vi "ClearWarning.vi"(9 "Error in":errorcluster) -> (1 "Error out":errorcluster)   [LabVIEW 2017, in "GPError.lvlib"]
doc: "Clears any warning on <B>Error in</B> but leaves any error.\n\nThis VI supports appended errors, clearing all warnings while leaving any errors.\n\nThis VI is inlined.\n\nSteen Schmidt\nGPower\n18/7 2013"
uses:
  GPError.lvlib
  Append/AppendMulti.vi
panel:
  # "Copyright © 2013\nSteen Schmidt, GPower\nSee enclosed license file for terms and conditions"
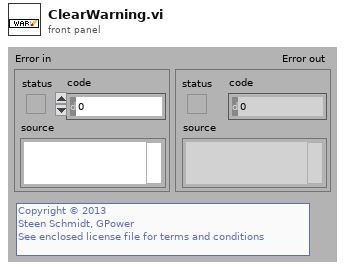
[diagram p1: front panel]
types:
  T1 = typedef "GPError.lvlib/ErrorType.ctl" = enum16{"No Error", "Error", "Warning", "Appended errors", "Appended warnings", "Appended mixed"}
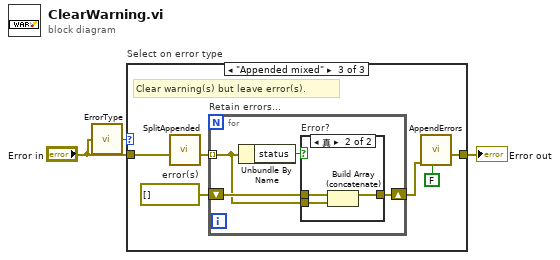
[diagram p0: block diagram]
diagram:
  n1 = call "ErrorType.vi"("Error in"="Error in") -> ("Error type"=w1:T1)  [unwired: 4 in]
  n2 = case "Select on error type" shown="\"Appended mixed\"" w1 {
    tunnel: "Error in" -> [w4 _ w10]
    tunnel: [w4 _ w6] -> w3
    frame "No Error", "Error", "Appended errors" {
      # "Leave 'No error' or error(s)."
    }
    frame "Warning", "Appended warnings" {
      # "Clear warning(s)."
    }
    frame "Appended mixed" {
      w8 = errorcluster[] []  # error(s)
      # "Clear warning(s) but leave error(s)."
      n3 = call "SplitAppended.vi"("Appended errors in"=w10) -> ("Errors out"=w9:errorcluster[])  [unwired: 10 in]
      n4 = for "Retain errors..." {
        tunnel: w9 -> [w12] mode=indexing
        shift-right: [w11] -> w7
        shift-left: w8 -> [w13]
        n5 = Unbundle By Name(w12) -> ("status"=w14:bool)
        n6 = case "Error?" shown="真" w14 {
          tunnel: w13 -> [w15 w18]
          tunnel: w12 -> [_ w17]
          tunnel: [w15 w16] -> w11
          frame False {
          }
          frame True {
            n7 = Build Array (concatenate)(w18, w17) -> (w16:errorcluster[])
          }
        }
      }
      n8 = call-poly "AppendErrors.vi"("Only append if new?"=FALSE, "Errors to append"=w7) -> ("Appended errors out"=w6:errorcluster)  [unwired: 9 in]
    }
  }
  "Error out" <- w3
